vi "Wärmepumpe.InitObject.vi"(8 "Error In":errorcluster, 11 "ModelMainPath":path) -> (0 "Error out":errorcluster, 3 "Wärmepumpe":refnum<data-value>)   [LabVIEW 2016, in "Wärmepumpe.lvclass"]
uses:
  Package ResourceControl/ObjectHandler/ObjectHandler.GetObjectWType.ctl
  Package ResourceControl/ObjectHandler/ObjectHandler.ObjectType.ctl
  Package ResourceControl/ObjectHandler/ObjectHandler.ObjectMessage.ctl
  Package ResourceControl/ObjectHandler/ObjectHandler.ObjectWType.ctl
  Package ResourceControl/ObjectHandler/ObjectHandler.lvclass
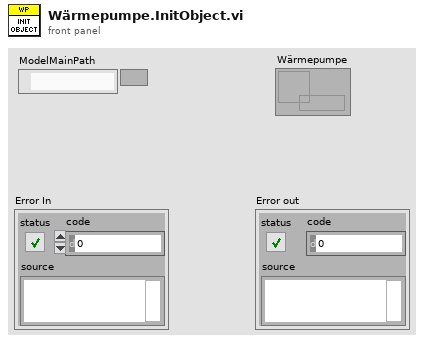
[diagram p1: front panel]
types:
  T1 = typedef "ObjectHandler.lvclass/ObjectHandler.ObjectMessage.ctl" = cluster{"Name":string, "ObjectWType":T2}
  T2 = typedef "ObjectHandler.lvclass/ObjectHandler.ObjectWType.ctl" = cluster{"ObjectType":T3, "Object":variant}
  T3 = typedef "ObjectHandler.lvclass/ObjectHandler.ObjectType.ctl" = enum16{"undefined", "ObjectHandler", "ViHandler", "ErrorHandler", "CentralStorage", "Hausmodell", "Sondenmodell", "Wärmepumpe", "Umgebung"}
  T4 = typedef "ObjectHandler.lvclass/ObjectHandler.GetObjectWType.ctl" = cluster{"Name":string, "Caller":string}
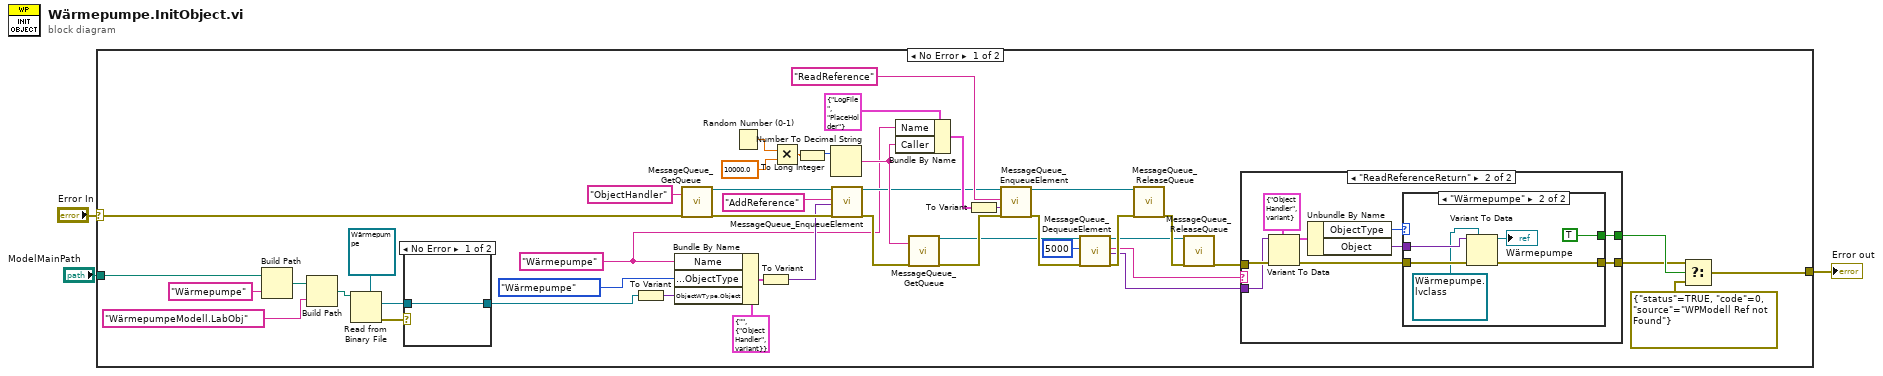
[diagram p0: block diagram]
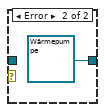
[diagram p2: hidden frame]
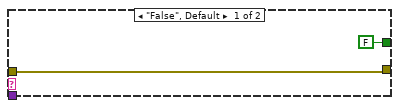
[diagram p3: hidden frame]
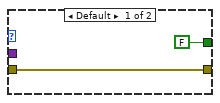
[diagram p4: hidden frame]
diagram:
  n1 = case shown="No Error" "Error In" {
    selector: "Error In" -> [w14 w71]
    tunnel: [w49 w71] -> w3
    tunnel: "ModelMainPath" -> [w4 _]
    frame No Error {
      w13 = "Wärmepumpe" ("Name")
      n2 = Build Path(base path=w4, name or relative path="Wärmepumpe") -> (appended path=w10:path)
      n3 = Build Path(base path=w10, name or relative path="WärmepumpeModell.LabObj") -> (appended path=w12:path)
      n4 = Read from Binary File(5:refnum<class "Wärmepumpe.lvclass"> refnum ("Wärmepumpe.lvclass"), 11:w12) -> (0:w8:errorcluster, 2:w7:refnum<class "Wärmepumpe.lvclass">)  [unwired: 4 in, 2 out]
      n5 = case shown="No Error" w8 {
        tunnel: [w50 refnum<class "Wärmepumpe.lvclass"> refnum ("Wärmepumpe.lvclass")] -> w5
        tunnel: w7 -> [w50 _]
        frame No Error {
        }
        frame Error {
        }
      }
      n6 = To Variant(anything=w5) -> (Variant=w21:variant)
      n7 = Bundle By Name(cluster=T1 {"Name"="", "ObjectWType"={"ObjectType"=enum."ObjectHandler", "Object"=variant(refnum<data-value> refnum)}} ("ObjectMessage"), "Name"=w13, "ObjectWType.ObjectType"=ObjectHandler.ObjectType."Wärmepumpe" ("ObjectType"), "ObjectWType.Object"=w21) -> (w20:T1)
      n8 = call "MessageQueue_GetQueue.vi"("Name"="ObjectHandler", "ErrorIn"=w14) -> ("QueueOut"=w23:refnum<queue>, "ErrorOut"=w24:errorcluster)  [unwired: 15 in, 1 out]
      n9 = Random Number (0-1)() -> (number: 0 to 1=w48:dbl)
      n10 = To Variant(anything=w20) -> (Variant=w19:variant)
      n11 = Multiply(x=w48, y=10000.0) -> (x*y=w46:dbl)
      n12 = To Long Integer(number=w46) -> (32bit integer=w45:i32)
      n13 = Number To Decimal String(number=w45) -> (decimal integer string=w30:string)  [unwired: 1 in]
      n14 = call "MessageQueue_EnqueueElement.vi"("QueueIn"=w23, "Message"="AddReference", "Data"=w19, "ErrorIn"=w24) -> ("QueueOut"=w15:refnum<queue>, "ErrorOut"=w16:errorcluster)  [unwired: 14 in]
      n15 = Bundle By Name(cluster=T4 {"Name"="LogFile", "Caller"="PlaceHolder"} ("GetRefInput"), "Name"=w13, "Caller"=w30) -> (w29:T4)
      n16 = call "MessageQueue_GetQueue.vi"("Name"=w30, "ErrorIn"=w16) -> ("QueueOut"=w39:refnum<queue>, "ErrorOut"=w44:errorcluster)  [unwired: 15 in, 1 out]
      n17 = To Variant(anything=w29) -> (Variant=w34:variant)
      n18 = call "MessageQueue_EnqueueElement.vi"("QueueIn"=w15, "Message"="ReadReference", "Data"=w34, "ErrorIn"=w44) -> ("QueueOut"=w40:refnum<queue>, "ErrorOut"=w43:errorcluster)  [unwired: 14 in]
      n19 = call "MessageQueue_DequeueElement.vi"("QueueIn"=w39, "Timeout"=5000, "ErrorIn"=w43) -> ("QueueOut"=w38:refnum<queue>, "Message"=w36:string, "Data"=w32:variant, "ErrorOut"=w42:errorcluster)  [unwired: 12 in, 1 out]
      n20 = call "MessageQueue_ReleaseQueue.vi"("QueueIn"=w40, "ErrorIn"=w42) -> ("ErrorOut"=w41:errorcluster)  [unwired: 15 in, 2 out]
      n21 = call "MessageQueue_ReleaseQueue.vi"("QueueIn"=w38, "ErrorIn"=w41) -> ("ErrorOut"=w33:errorcluster)  [unwired: 15 in, 2 out]
      n22 = case shown="\"ReadReferenceReturn\"" w36 {
        tunnel: w33 -> [w52 w62]
        tunnel: w32 -> [_ w61]
        tunnel: [w52 w55] -> w27
        tunnel: [FALSE w54] -> w28
        frame "False", Default {
        }
        frame "ReadReferenceReturn" {
          n23 = Variant To Data(error in=w62, type=T2 {"ObjectType"=enum."ObjectHandler", "Object"=variant} ("ObjectWType"), Variant=w61) -> (data=w59:T2, error out=w56:errorcluster)
          n24 = Unbundle By Name(w59) -> ("ObjectType"=w58:T3, "Object"=w57:variant)
          n25 = case shown="\"Wärmepumpe\"" w58 {
            tunnel: w57 -> [_ w70]
            tunnel: w56 -> [w64 w69]
            tunnel: [w64 w68] -> w55
            tunnel: [FALSE TRUE] -> w54
            frame Default {
            }
            frame "Wärmepumpe" {
              n26 = Variant To Data(error in=w69, type=refnum<data-value> refnum ("data value reference"), Variant=w70) -> (data=→"Wärmepumpe":refnum<data-value>, error out=w68:errorcluster)
            }
          }
        }
      }
      n27 = Select(t=w27, s=w28, f=errorcluster {"status"=TRUE, "code"=0, "source"="WPModell Ref not Found"}) -> (s? t:f=w49:errorcluster)
    }
    frame Error {
    }
  }
  "Error out" <- w3
